vi "Evaluate Partial Derivatives of 1-Exp.vi"(8 "error in (no error)":errorcluster, 9 "Ramp":dbl[](array[numeric]), 10 "Fitted Parameter Names":T2[](array[typedef]), 11 "Exp Parameters":T3) -> (0 "error out":errorcluster, 3 "Partial Derivatives Plot Array":T1[](array[typedef]))   [LabVIEW 2021, in "Fits.lvlib"]
uses:
  Fits.lvlib
  1-Exp Parameters.ctl
  IRF(X)PSED/Decay Fit Parameters In List.ctl
  Graphs/XY Graph/XY Graph Plot Data.ctl
  3a6f6af8-dfdd-45d2-a48b-969f03fc1cd8.vi
  Graphs/XY Graph/XY Graph Add-Ons.lvlib
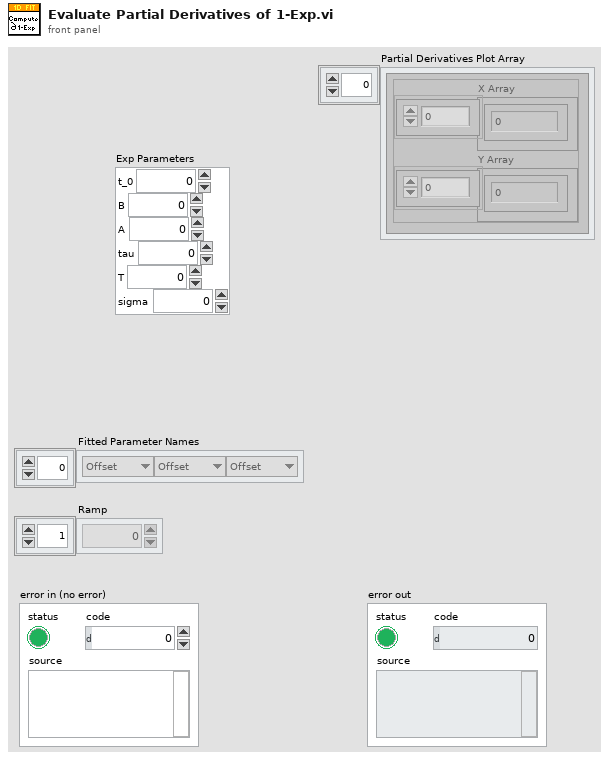
[diagram p1: front panel]
types:
  T1 = typedef "XY Graph Add-Ons.lvlib/XY Graph Plot Data.ctl" = cluster{"X Array":dbl[], "Y Array":dbl[]}
  T2 = typedef "Fits.lvlib/Decay Fit Parameters In List.ctl" = enum16{"Offset", "Baseline", "A_1", "tau_1", "A_2", "tau_2"}
  T3 = typedef "Fits.lvlib/1-Exp Parameters.ctl" = cluster{"t_0":dbl, "B":dbl, "A":dbl, "tau":dbl, "T":dbl, "sigma":dbl}
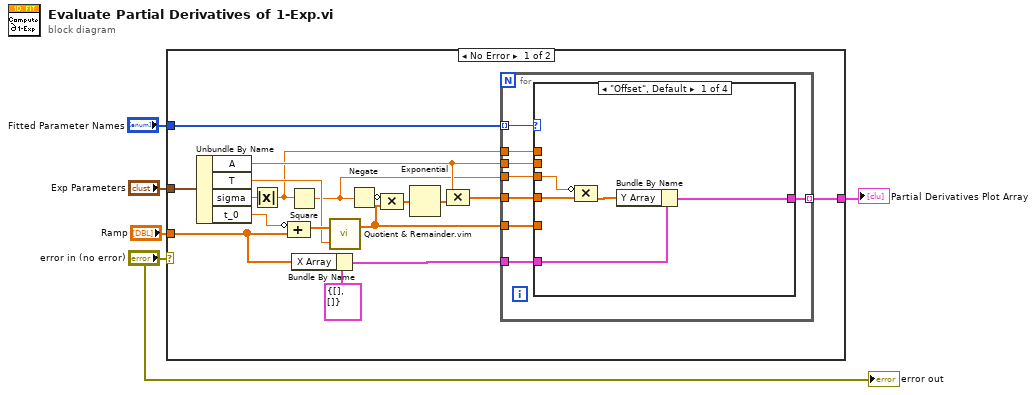
[diagram p0: block diagram]
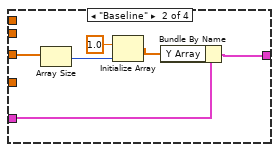
[diagram p2: hidden frame]
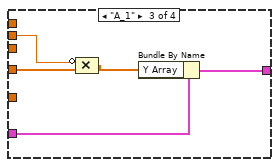
[diagram p3: hidden frame]
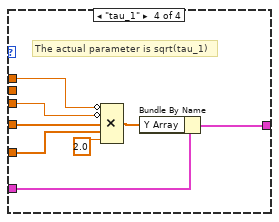
[diagram p4: hidden frame]
diagram:
  n1 = case shown="No Error" "error in (no error)" {
    tunnel: "Exp Parameters" -> [w23 _]
    tunnel: "Ramp" -> [w15 _]
    tunnel: "Fitted Parameter Names" -> [w16 _]
    tunnel: [w9 _] -> w1
    frame No Error {
      n2 = Unbundle By Name(w23) -> ("A"=w8:dbl, "T"=w20:dbl, "sigma"=w11:dbl, "t_0"=w22:dbl)
      n3 = Absolute Value(x=w11) -> (abs(x)=w6:dbl)
      n4 = Compound Arithmetic op=ADD(invert w22, w15) -> (w21:dbl[])
      n5 = Square(x=w6) -> (x^2=w7:dbl)
      n6 = Bundle By Name(cluster=T1 {"X Array"=[], "Y Array"=[]} ("Plot"), "X Array"=w15) -> (w13:T1)
      n7 = call "Quotient & Remainder.vim"("y"=w20, "x"=w21) -> ("x - E(x/y)y"=w10:dbl[])  [unwired: 1 out]
      n8 = Negate(x=w7) -> (-x=w17:dbl)
      n9 = Compound Arithmetic op=MULTIPLY(invert w17, w10) -> (w19:dbl[])
      n10 = Exponential(1:w19) -> (0:w18:dbl[])
      n11 = Compound Arithmetic op=MULTIPLY(w8, w18) -> (w12:dbl[])
      n12 = for {
        tunnel: w16 -> [w31] mode=indexing
        tunnel: w13 -> [w30]
        tunnel: w12 -> [w29]
        tunnel: w7 -> [w28]
        tunnel: w10 -> [w27]
        tunnel: [w26] -> w9 mode=indexing
        tunnel: w8 -> [w25]
        tunnel: w6 -> [w24]
        n13 = case shown="\"Offset\", Default" w31 {
          tunnel: w30 -> [w33 w37 w45 w53]
          tunnel: w29 -> [w36 w42 w47 w55]
          tunnel: w28 -> [w35 _ _ w49]
          tunnel: [w32 w38 w44 w51] -> w26
          tunnel: w27 -> [_ _ _ w54]
          tunnel: w25 -> [_ _ w43 _]
          tunnel: w24 -> [_ _ _ w48]
          frame "Offset", Default {
            n14 = Compound Arithmetic op=MULTIPLY(invert w35, w36) -> (w34:dbl[])
            n15 = Bundle By Name(cluster=w33, "Y Array"=w34) -> (w32:T1)
          }
          frame "Baseline" {
            n16 = Array Size(array=w42) -> (size(s)=w41:i32)
            n17 = Initialize Array(1.0 ("element"), w41) -> (w39:dbl[])
            n18 = Bundle By Name(cluster=w37, "Y Array"=w39) -> (w38:T1)
          }
          frame "A_1" {
            n19 = Compound Arithmetic op=MULTIPLY(invert w43, w47) -> (w46:dbl[])
            n20 = Bundle By Name(cluster=w45, "Y Array"=w46) -> (w44:T1)
          }
          frame "tau_1" {
            # "The actual parameter is sqrt(tau_1)"
            n21 = Compound Arithmetic op=MULTIPLY(invert w48, invert w49, w55, w54, 2.0) -> (w52:dbl[])
            n22 = Bundle By Name(cluster=w53, "Y Array"=w52) -> (w51:T1)
          }
        }
      }
    }
    frame Error {
    }
  }
  "Partial Derivatives Plot Array" <- w1
  "error out" <- "error in (no error)"
